vi "Initialise.vi"(8 "error in (no error)":errorcluster, 11 "Node in":refnum<class "bt_Send_Queue.lvclass">) -> (0 "error out":errorcluster, 3 "Node out":refnum<class "bt_Send_Queue.lvclass">)   [LabVIEW 2021, in "BT.lvlib" / "bt_Send_Queue.lvclass"]
uses:
  bt_Send_Queue.lvclass
  bt_Send_Queue.lvclass/bt_Send_Queue.ctl
  With Values/Send/bt_Send_Synch_WithValues.lvclass
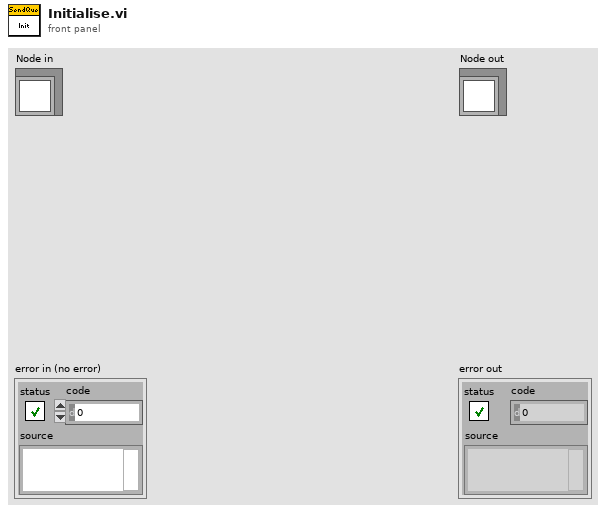
[diagram p1: front panel]
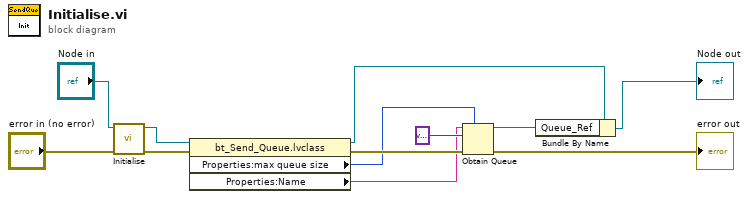
[diagram p0: block diagram]
diagram:
  n1 = call-parent "Initialise.vi"("error in (no error)"="error in (no error)", "Node in"="Node in") -> ("error out"=w6:errorcluster, "Node out"=w5:refnum<class "bt_Send_Queue.lvclass">)  [unwired: 8 in]
  n2 = property class="bt_Send_Queue.lvclass"(reference=w5, error in=w6) -> (reference out=w4:refnum<class "bt_Send_Queue.lvclass">, error out=w3:errorcluster, "Properties:max queue size"=w2:i32, "Properties:Name"=w1:string)
  n3 = Obtain Queue(max queue size (-1, unlimited)=w2, name (unnamed)=w1, element data type=variant, error in (no error)=w3) -> (queue out=w9:refnum<queue>, error out=→"error out":errorcluster)  [unwired: 1 in, 1 out]
  n4 = Bundle By Name(cluster=w4, "Queue_Ref"=w9) -> (→"Node out":refnum<class "bt_Send_Queue.lvclass">)
